vi "parse_lidar_configuration.vi"(3 "error in":errorcluster, 5 "Lidar configuration":string) -> (0 "error out":errorcluster, 1 "Number points":i32, 2 "Number packets":i32)   [LabVIEW 2019]
doc: "Calculates the number of packets and the number of points in a LiDAR stream based on the horizontal resolution."
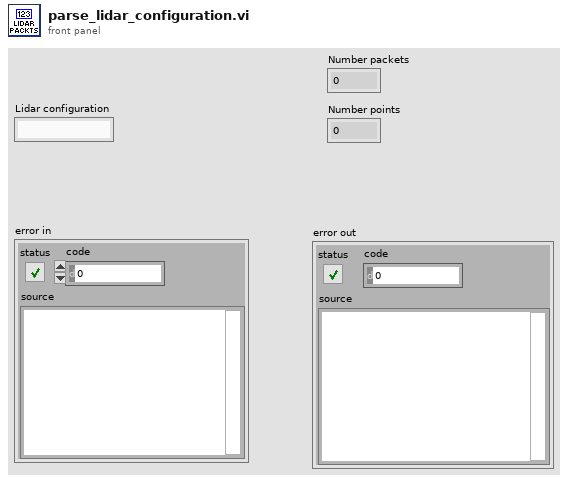
[diagram p1: front panel]
types:
  T1 = cluster{"horizontal_resolution":dbl, "n_lasers":i32}
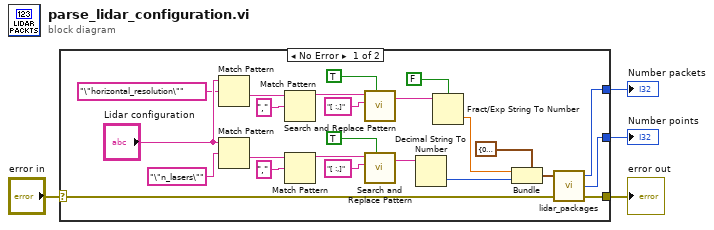
[diagram p0: block diagram]
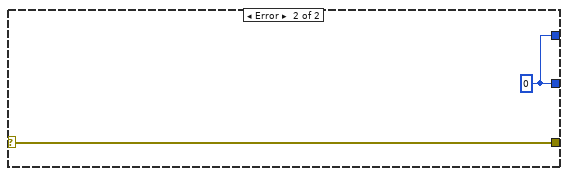
[diagram p2: hidden frame]
diagram:
  n1 = case shown="No Error" "error in" {
    selector: "error in" -> [w8 w30]
    tunnel: [w7 w30] -> w3
    tunnel: [w6 w29] -> w2
    tunnel: [w5 w29] -> w1
    frame No Error {
      n2 = Match Pattern(string="Lidar configuration", regular expression="\"horizontal_resolution\"") -> (after substring=w12:string)  [unwired: 1 in, 3 out]
      n3 = Match Pattern(string="Lidar configuration", regular expression="\"n_lasers\"") -> (after substring=w20:string)  [unwired: 1 in, 3 out]
      n4 = Match Pattern(string=w12, regular expression=",") -> (before substring=w14:string)  [unwired: 1 in, 3 out]
      n5 = Match Pattern(string=w20, regular expression=",") -> (before substring=w16:string)  [unwired: 1 in, 3 out]
      n6 = call <vilib>:"Search and Replace Pattern.vi"("string"=w14, "regular expression (\"\")"="[ :,]" ("regular expression (\"\")"), "replace all? (F)"=TRUE) -> ("result string"=w21:string)  [unwired: 2 in, 1 out]
      n7 = call <vilib>:"Search and Replace Pattern.vi"("string"=w16, "regular expression (\"\")"="[ :,]" ("regular expression (\"\")"), "replace all? (F)"=TRUE) -> ("result string"=w22:string)  [unwired: 2 in, 1 out]
      n8 = Decimal String To Number(string=w22) -> (number=w24:i32)  [unwired: 2 in, 1 out]
      n9 = Fract/Exp String To Number(use system decimal point (T)=FALSE, string=w21) -> (number=w23:dbl)  [unwired: 2 in, 1 out]
      n10 = Bundle(cluster=T1 {"horizontal_resolution"=0.0, "n_lasers"=0}, "horizontal_resolution"=w23, "n_lasers"=w24) -> (w26:T1)
      n11 = call "lidar_packages.vi"("error in"=w8, "Settings"=w26) -> ("error out"=w7:errorcluster, "Number points"=w6:i32, "Packets"=w5:i32)  [unwired: 1 in]
    }
    frame Error {
      w29 = 0 ("packets")
    }
  }
  "error out" <- w3
  "Number points" <- w2
  "Number packets" <- w1
